vi "TDC_DAQV23_Paralled_muon.vi"(8 "error in (no error)":errorcluster, 9 "stop":bool, 10 "save data":bool=TRUE, 11 "SMA mode":bool) -> (3 "rate":dbl=15.40764551745953)   [LabVIEW 2017]
uses:
  <vilib>/Utility/file.llb/Write Delimited Spreadsheet (DBL).vi
  <vilib>/Utility/file.llb/Write Delimited Spreadsheet (I64).vi
panel:
  out "name (unnamed)":string
  out "x+y":u64
  out "ip":string[](array[string])
  out "error out 4":errorcluster
  in  "timeout (ms) 2":i32=10000
  in  "address":string[](array[string])=["192.168.10.23", "192.168.10.21"]
  out "substring 4":string
  out "substring 3":string
  out "hex integer string":string="07E8"
  out "Year":string="2024"
  out "substring 2":string
  out "substring":string
  in  "factor":i32=128
  in  "displayCR":bool=TRUE
  in  "Counter Setting":dbl=100000.0 format="%#_13g"
  in  "replace dat":bool
  in  "append csv":bool=TRUE
  out "number":u32=23
  out "element":string
  out "fine":u64=375 format="%x"
  in  "UDP Config":bool=TRUE
  in  "data  path":path=path "G:/tdc/2017"
  out "cal 2":u64[](graph)
  in  "Thresholds (mV)":u16[](array[numeric])=[580, 580, 580, 580, 600, 600, 600, 600, 580, 580, 600, 600, 600, 600, 600, 600, 580, 580, 600, 600, 600, 600, 600, 600, 580, 580, 600, 600, 600, 600, 600, 600]
  out "error out 2":errorcluster={"status"=TRUE, "code"=1, "source"="Dequeue Element in TDC_DAQV18_NewStructure.vi"}
  in  "display":bool=TRUE
  in  "Thresholds":u16=580
  in  "one key for threshold":bool=TRUE
  in  "RST":bool
  in  "通道数量":i32=64
  out "Cal Table":u32[](array[numeric])=[33400, 33400, 0, 0, 0, 0, 0, 0, 0, 0, 0, 0, 0, 0, 0, 0, 0, 0, 0, 0, 0, 0, 0, 0, 0, 0, 0, 0, 0, 0, 0, 0, 0, 0, 0, 0, 0, 0, 0, 0, 0, 0, 0, 0, 0, 0, 0, 0, 0, 0, 0, 0, 0, 0, 0, 0, 0, 0, 0, 0, 0, 0, 0, 0]
  in  "channel for cal":i32
  out "channel number":u64=1
  out "Calibration Counter":i32=33403
  out "cal":u32[](graph)=[0, 0, 0, 0, 0, 0, 0, 0, 0, 0, 0, 0, 0, 0, 0, 0, 0, 0, 0, 0, 0, 0, 0, 0, 0, 0, 0, 0, 0, 0, 0, 0, 0, 0, 0, 0, 0, 0, 0, 0, 0, 0, 0, 0, 0, 0, 0, 0, 0, 0, 0, 0, 0, 0, 0, 0, 0, 0, 0, 0, 0, 0, 0, 0, 0, 0, 0, 0, 0, 0, 0, 0, 0, 0, 0, 0, 0, 0, 0, 0, 0, 0, 0, 0, 0, 0, 0, 0, 0, 0, 0, 0, 0, 0, 0, 0, 0, 0, 0, 0, 0, 0, 0, 0, 0, 0, 0, 0, 0, 0, 0, 0, 0, 0, 0, 0, 0, 0, 0, 0, 0, 0, 0, 0, 0, 0, 0, 0, 0, 0, 0, 0, 0, 0, 0, 0, 0, 0, 0, 0, 0, 0, 0, 0, 0, 0, 0, 0, 0, 0, 0, 0, 0, 0, 0, 0, 0, 0, 0, 0, 0, 0, 0, 0, 0, 0, 0, 0, 0, 0, 0, 0, 0, 0, 0, 0, 0, 0, 0, 0, 0, 0, 0, 0, 0, 0, 0, 0, 0, 0, 0, 0, 0, 0, 0, 0, 0, 0, 0, 0, 0, 0, 0, 0, 0, 0, 0, 0, 0, 0, 0, 0, 0, 0, 0, 0, 0, 0, 0, 0, 0, 0, 0, 0, 0, 0, 0, 0, 0, 0, 0, 0, 0, 0, 0, 0, 0, 0, 0, 0, 0, 6, 23, 55, 10, 109, 60, 9, 21, 55, 21, 185, 19, 80, 25, 73, 17, 22, 36, 28, 37, 99, 26, 26, 64, 113, 69, 7, 14, 18, 136, 20, 15, 79, 14, 27, 31, 33, 186, 15, 16, 24, 85, 10, 20, 164, 11, 7, 26, 8, 56, 214, 23, 59, 6, 25, 14, 93, 49, 18, 107, 57, 21, 11, 76, 16, 93, 28, 118, 65, 51, 32, 70, 13, 49, 31, 28, 95, 11, 61, 50, 18, 12, 25, 16, 21, 25, 65, 81, 19, 18, 21, 52, 13, 66, 54, 29, 13, 105, 14, 26, 25, 16, 98, 16, 6, 117, 40, 58, 73, 32, 16, 42, 15, 24, 43, 27, 78, 34, 19, 9, 22, 13, 13, 78, 25, 34, 17, 35, 62, 14, 60, 11, 26, 6, 12, 18, 8, 36, 37, 14, 15, 77, 16, 72, 14, 8, 24, 30, 36, 38, 215, 11, 17, 25, 7, 37, 58, 189, 49, 13, 12, 8, 5, 88, 13, 20, 23, 139, 18, 18, 30, 10, 17, 25, 26, 77, 71, 13, 18, 10, 62, 11, 17, 32, 14, 33, 69, 23, 23, 23, 147, 25, 21, 19, 88, 29, 15, 28, 12, 4, 12, 127, 66, 25, 73, 13, 11, 6, 16, 69, 32, 14, 27, 34, 118, 16, 11, 8, 12, 35, 58, 21, 15, 45, 150, 15, 54, 14, 20, 7, 16, 55, 24, 45, 93, 87, 11, 17, 9, 113, 11, 15, 104, 62, 38, 84, 27, 8, 8, 62, 95, 42, 49, 45, 111, 29, 50, 80, 19, 26, 15, 37, 142, 29, 80, 36, 14, 12, 114, 28, 15, 13, 70, 57, 13, 7, 47, 46, 92, 84, 75, 19, 165, 62, 8, 25, 63, 59, 65, 23, 97, 20, 11, 86, 12, 36, 24, 96, 19, 7, 20, 29, 66, 43, 31, 80, 23, 20, 52, 15, 79, 19, 13, 30, 18, 14, 11, 17, 119, 19, 97, 11, 14, 31, 15, 87, 17, 127, 47, 23, 15, 64, 11, 19, 14, 24, 46, 60, 62, 65, 13, 37, 16, 17, 23, 55, 41, 48, 15, 30, 69, 30, 130, 58, 13, 27, 22, 25, 86, 13, 107, 31, 29, 12, 25, 31, 32, 16, 31, 20, 42, 30, 2, 57, 37, 34, 16, 28, 40, 42, 14, 90, 51, 22, 91, 31, 22, 103, 20, 9, 19, 127, 40, 39, 10, 22, 13, 11, 60, 52, 17, 44, 70, 25, 58, 12, 40, 43, 30, 29, 39, 120, 23, 12, 15, 40, 5, 44, 16, 29, 21, 79, 15, 28, 83, 67, 17, 19, 109, 14, 21, 7, 23, 19, 48, 17, 24, 62, 95, 15, 28, 43, 190, 39, 94, 24, 18, 19, 78, 117, 18, 22, 28, 92, 13, 17, 71, 20, 43, 15, 99, 10, 14, 15, 67, 65, 17, 20, 90, 42, 16, 25, 79, 7, 12, 14, 41, 15, 30, 24, 183, 25, 20, 14, 19, 80, 10, 18, 135, 40, 100, 17, 25, 134, 82, 7, 103, 25, 59, 27, 107, 32, 48, 68, 13, 13, 33, 67, 60, 38, 74, 29, 14, 16, 10, 51, 19, 47, 39, 134, 33, 47, 25, 56, 34, 12, 116, 51, 11, 10, 36, 18, 29, 13, 14, 84, 13, 54, 43, 13, 43, 39, 51, 32, 46, 8, 15, 16, 66, 40, 10, 30, 151, 15, 7, 117, 23, 17, 49, 12, 28, 42, 76, 45, 15, 25, 72, 8, 8, 13, 18, 59, 52, 13, 13, 19, 64, 10, 27, 51, 8, 19, 13, 40, 128, 32, 129, 26, 177, 23, 10, 20, 27, 71, 70, 17, 19, 23, 30, 48, 33, 38, 51, 88, 20, 38, 27, 36, 8, 9, 14, 4, 70, 27, 110, 31, 25, 33, 66, 49, 34, 41, 108, 42, 15, 95, 32, 72, 31, 23, 51, 124, 31, 28, 20, 129, 11, 14, 52, 152, 13, 124, 108, 52, 43, 20, 78, 18, 82, 20, 74, 19, 46, 13, 30, 73, 47, 71, 18, 32, 54, 17, 11, 13, 28, 47, 130, 21, 25, 26, 40, 34, 28, 31, 12, 51, 21, 161, 11, 5, 6, 25, 16, 19, 23, 44, 98, 35, 54, 11, 21, 67, 42, 69, 5, 5, 19, 14, 14, 132, 14, 42, 81, 23, 21, 83, 13, 8, 81, 29, 108, 20, 16, 33, 130, 18, 50, 22, 15, 12, 51, 125, 13, 15, 34, 24, 19, 65, 21, 18, 68, 39, 19, 22, 59, 18, 12, 24, 55, 20, 39, 73, 14, 12, 58, 89, 37, 106, 64, 14, 17, 11, 69, 29, 122, 28, 13, 11, 53, 23, 12, 85, 24, 19, 95, 3, 20, 12, 41, 18, 21, 34, 57, 48, 26, 36, 64, 45, 42, 78, 3, 26, 31, 19, 110, 36, 37, 23, 52, 30, 24, 24, 61, 22, 19, 36, 23, 60, 12, 17, 50, 33, 37, 68, 25, 23, 14, 14, 26, 23, 26, 0, 4, 5, 6, 0, 0, 0, 0, 0, 0, 0, 0, 0, 0, 0, 0, 0, 0, 0, 0, 0, 0, 0, 0, 0, 0, 0, 0, 0, 0, 0, 0, 0, 0, 0, 0, 0, 0, 0, 0, 0, 0, 0, 0, 0, 0, 0, 0, 0, 0, 0, 0, 0, 0, 0, 0, 0, 0, 0, 0, 0, 0, 0, 0, 0, 0, 0, 0, 0, 0, 0, 0, 0, 0, 0, 0, 0, 0, 0, 0, 0, 0, 0, 0, 0, 0, 0, 0, 0, 0, 0, 0, 0, 0, 0, 0, 0, 0, 0, 0, 0, 0, 0, 0, 0, 0, 0, 0, 0, 0, 0, 0, 0, 0, 0, 0, 0, 0, 0, 0, 0, 0, 0, 0, 0, 0, 0, 0, 0, 0, 0, 0, 0, 0, 0, 0, 0, 0, 0, 0, 0, 0, 0, 0, 0, 0, 0, 0, 0, 0, 0, 0, 0, 0, 0, 0, 0, 0, 0, 0, 0, 0, 0, 0, 0, 0, 0, 0, 0, 0, 0, 0, 0, 0, 0, 0, 0, 0, 0, 0, 0, 0, 0, 0, 0, 0, 0, 0, 0, 0, 0, 0, 0, 0, 0, 0, 0, 0, 0, 0, 0, 0, 0, 0, 0, 0, 0, 0, 0, 0, 0, 0, 0, 0, 0, 0, 0, 0, 0, 0, 0, 0, 0, 0, 0, 0, 0, 0, 0, 0, 0, 0, 0, 0, 0, 0, 0, 0, 0, 0, 0, 0, 0, 0, 0, 0, 0, 0, 0, 0, 0, 0, 0, 0, 0, 0, 0, 0, 0, 0, 0, 0, 0, 0, 0, 0, 0, 0, 0, 0, 0, 0, 0, 0, 0, 0, 0, 0, 0, 0, 0, 0, 0, 0, 0, 0, 0, 0, 0, 0, 0, 0, 0, 0, 0, 0, 0, 0, 0, 0, 0, 0, 0, 0, 0, 0, 0, 0, 0, 0, 0, 0, 0, 0, 0, 0, 0, 0, 0, 0, 0, 0, 0, 0, 0, 0, 0, 0, 0, 0, 0, 0, 0, 0, 0, 0, 0, 0, 0, 0, 0, 0, 0, 0, 0, 0, 0, 0, 0, 0, 0, 0, 0, 0, 0, 0, 0, 0, 0, 0, 0, 0, 0, 0, 0, 0, 0, 0, 0, 0, 0, 0, 0, 0, 0, 0, 0, 0, 0, 0, 0, 0, 0, 0, 0, 0, 0, 0, 0, 0, 0, 0, 0, 0, 0, 0, 0, 0, 0, 0, 0, 0, 0, 0, 0, 0, 0, 0, 0, 0, 0, 0, 0, 0, 0, 0, 0, 0, 0, 0, 0, 0, 0, 0, 0, 0, 0, 0, 0, 0, 0, 0, 0, 0, 0, 0, 0, 0, 0, 0, 0, 0, 0, 0, 0, 0, 0, 0, 0, 0, 0, 0, 0, 0, 0, 0, 0, 0, 0, 0, 0, 0, 0, 0, 0, 0, 0, 0, 0, 0, 0, 0, 0, 0, 0, 0, 0, 0, 0, 0, 0, 0, 0, 0, 0, 0, 0, 0, 0, 0, 0, 0, 0, 0, 0, 0, 0, 0, 0, 0, 0, 0, 0, 0, 0, 0, 0, 0, 0, 0, 0, 0, 0, 0, 0, 0, 0, 0, 0, 0, 0, 0, 0, 0, 0, 0, 0, 0, 0, 0, 0, 0, 0, 0, 0, 0, 0, 0, 0, 0, 0, 0, 0, 0, 0, 0, 0, 0, 0, 0, 0, 0, 0, 0, 0, 0, 0, 0, 0, 0, 0, 0, 0, 0, 0, 0, 0, 0, 0, 0, 0, 0, 0, 0, 0, 0, 0, 0, 0, 0, 0, 0, 0, 0, 0, 0, 0, 0, 0, 0, 0, 0, 0, 0, 0, 0, 0, 0, 0, 0, 0, 0, 0, 0, 0, 0, 0, 0, 0, 0, 0, 0, 0, 0, 0, 0, 0, 0, 0, 0, 0, 0, 0, 0, 0, 0, 0, 0, 0, 0, 0, 0, 0, 0, 0, 0, 0, 0, 0, 0, 0, 0, 0, 0, 0, 0, 0, 0, 0, 0, 0, 0, 0, 0, 0, 0, 0, 0, 0, 0, 0, 0, 0, 0, 0, 0, 0, 0, 0, 0, 0, 0, 0, 0, 0, 0, 0, 0, 0, 0, 0, 0, 0, 0, 0, 0, 0, 0, 0, 0, 0, 0, 0, 0, 0, 0, 0, 0, 0, 0, 0, 0, 0, 0, 0, 0, 0, 0, 0, 0, 0, 0, 0, 0, 0, 0, 0, 0, 0, 0, 0, 0, 0, 0, 0, 0, 0, 0, 0, 0, 0, 0, 0, 0, 0, 0, 0, 0, 0, 0, 0, 0, 0, 0, 0, 0, 0, 0, 0, 0, 0, 0, 0, 0, 0, 0, 0, 0, 0, 0, 0, 0, 0, 0, 0, 0, 0, 0, 0, 0, 0, 0, 0, 0, 0, 0, 0, 0, 0, 0, 0, 0, 0, 0, 0, 0, 0, 0, 0, 0, 0, 0, 0, 0, 0, 0, 0, 0, 0, 0, 0, 0, 0, 0, 0, 0, 0, 0, 0, 0, 0, 0, 0, 0, 0, 0, 0, 0, 0, 0, 0, 0, 0, 0, 0, 0, 0, 0, 0, 0, 0, 0, 0, 0, 0, 0, 0, 0, 0, 0, 0, 0, 0, 0, 0, 0, 0, 0, 0, 0, 0, 0, 0, 0, 0, 0, 0, 0, 0, 0, 0, 0, 0, 0, 0, 0, 0, 0, 0, 0, 0, 0, 0, 0, 0, 0, 0, 0, 0, 0, 0, 0, 0, 0, 0, 0, 0, 0, 0, 0, 0, 0, 0, 0, 0, 0, 0, 0, 0, 0, 0, 0, 0, 0, 0, 0, 0, 0, 0, 0, 0, 0, 0, 0, 0, 0, 0, 0, 0, 0, 0, 0, 0, 0, 0, 0, 0, 0, 0, 0, 0, 0, 0, 0, 0, 0, 0, 0, 0, 0, 0, 0, 0, 0, 0, 0, 0, 0, 0, 0, 0, 0, 0, 0, 0, 0, 0, 0, 0, 0, 0, 0, 0, 0, 0, 0, 0, 0, 0, 0, 0, 0, 0, 0, 0, 0, 0, 0, 0, 0, 0, 0, 0, 0, 0, 0, 0, 0, 0, 0, 0, 0, 0, 0, 0, 0]
  out "error out":errorcluster
  out "appended path":path=path "G:/tdc/2017/test_20240929_011527.dat"
  in  "filename":string="test"
  in  "Events":i32=110000 min=1
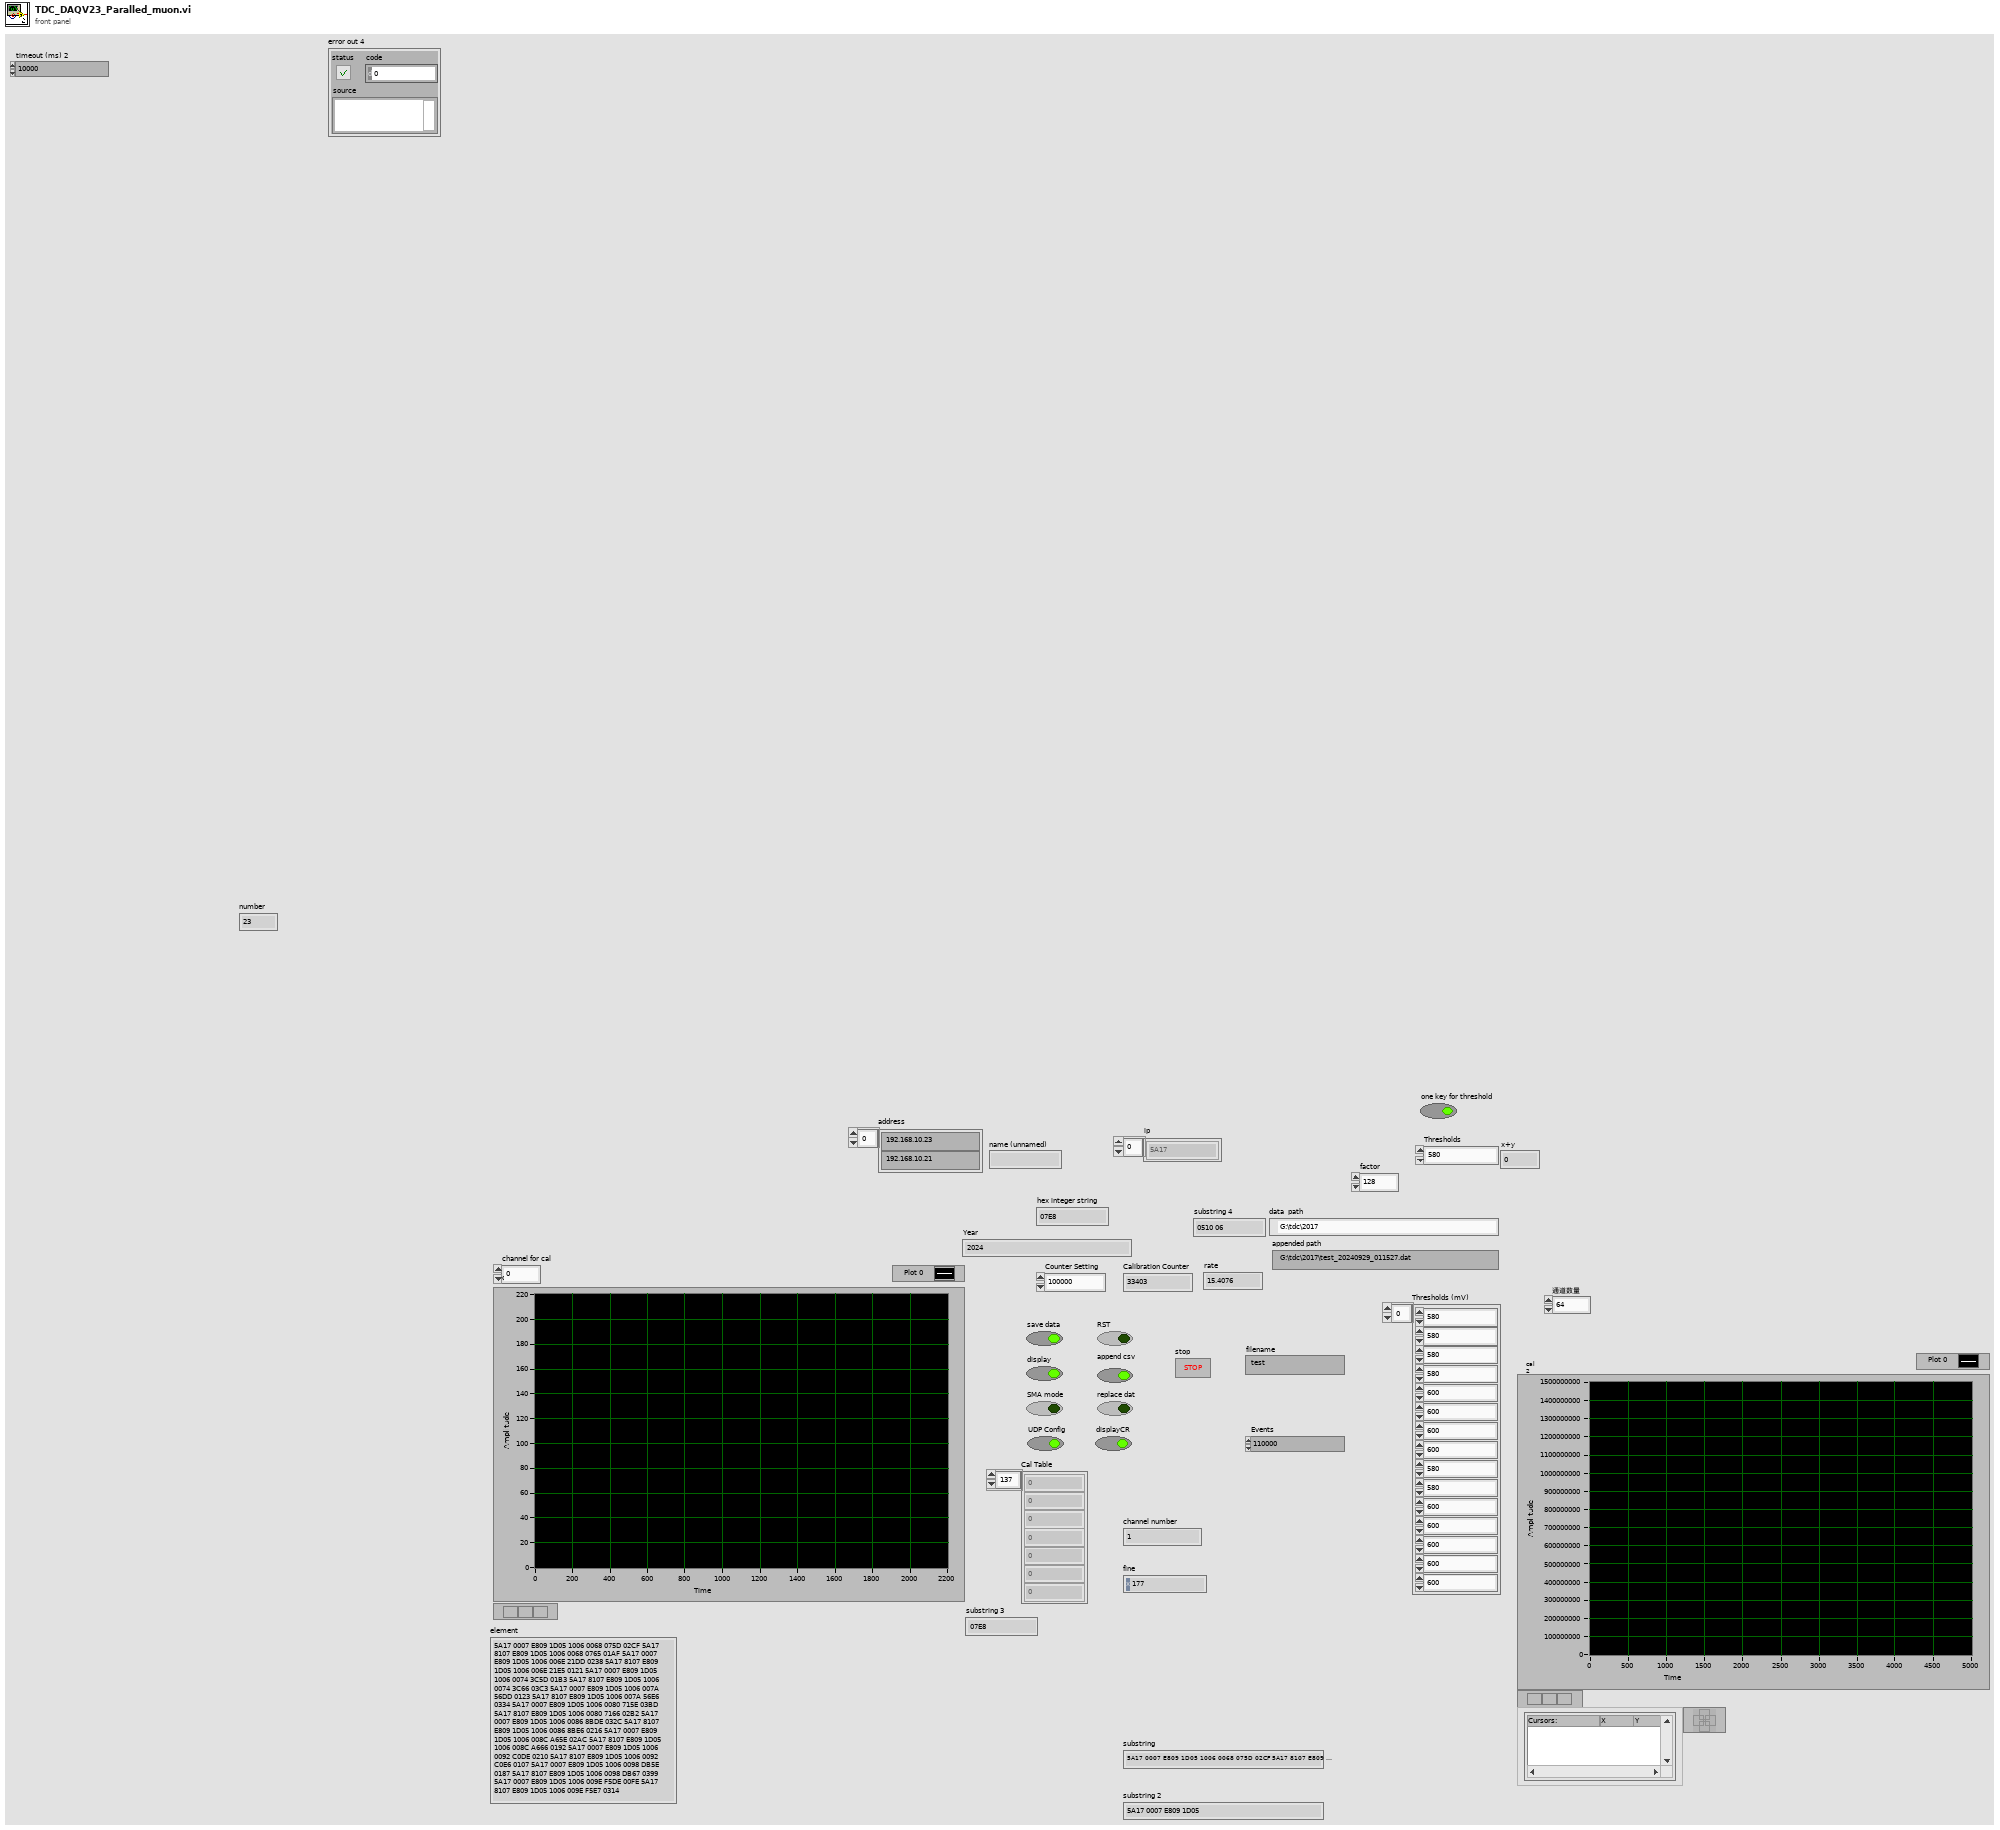
[diagram p1: front panel]
types:
  T1 = enum16{"open", "replace", "create", "open or create", "replace or create", "replace or create with confirmation"}
  T2 = enum16{"big-endian, network order", "native, host order", "little-endian"}
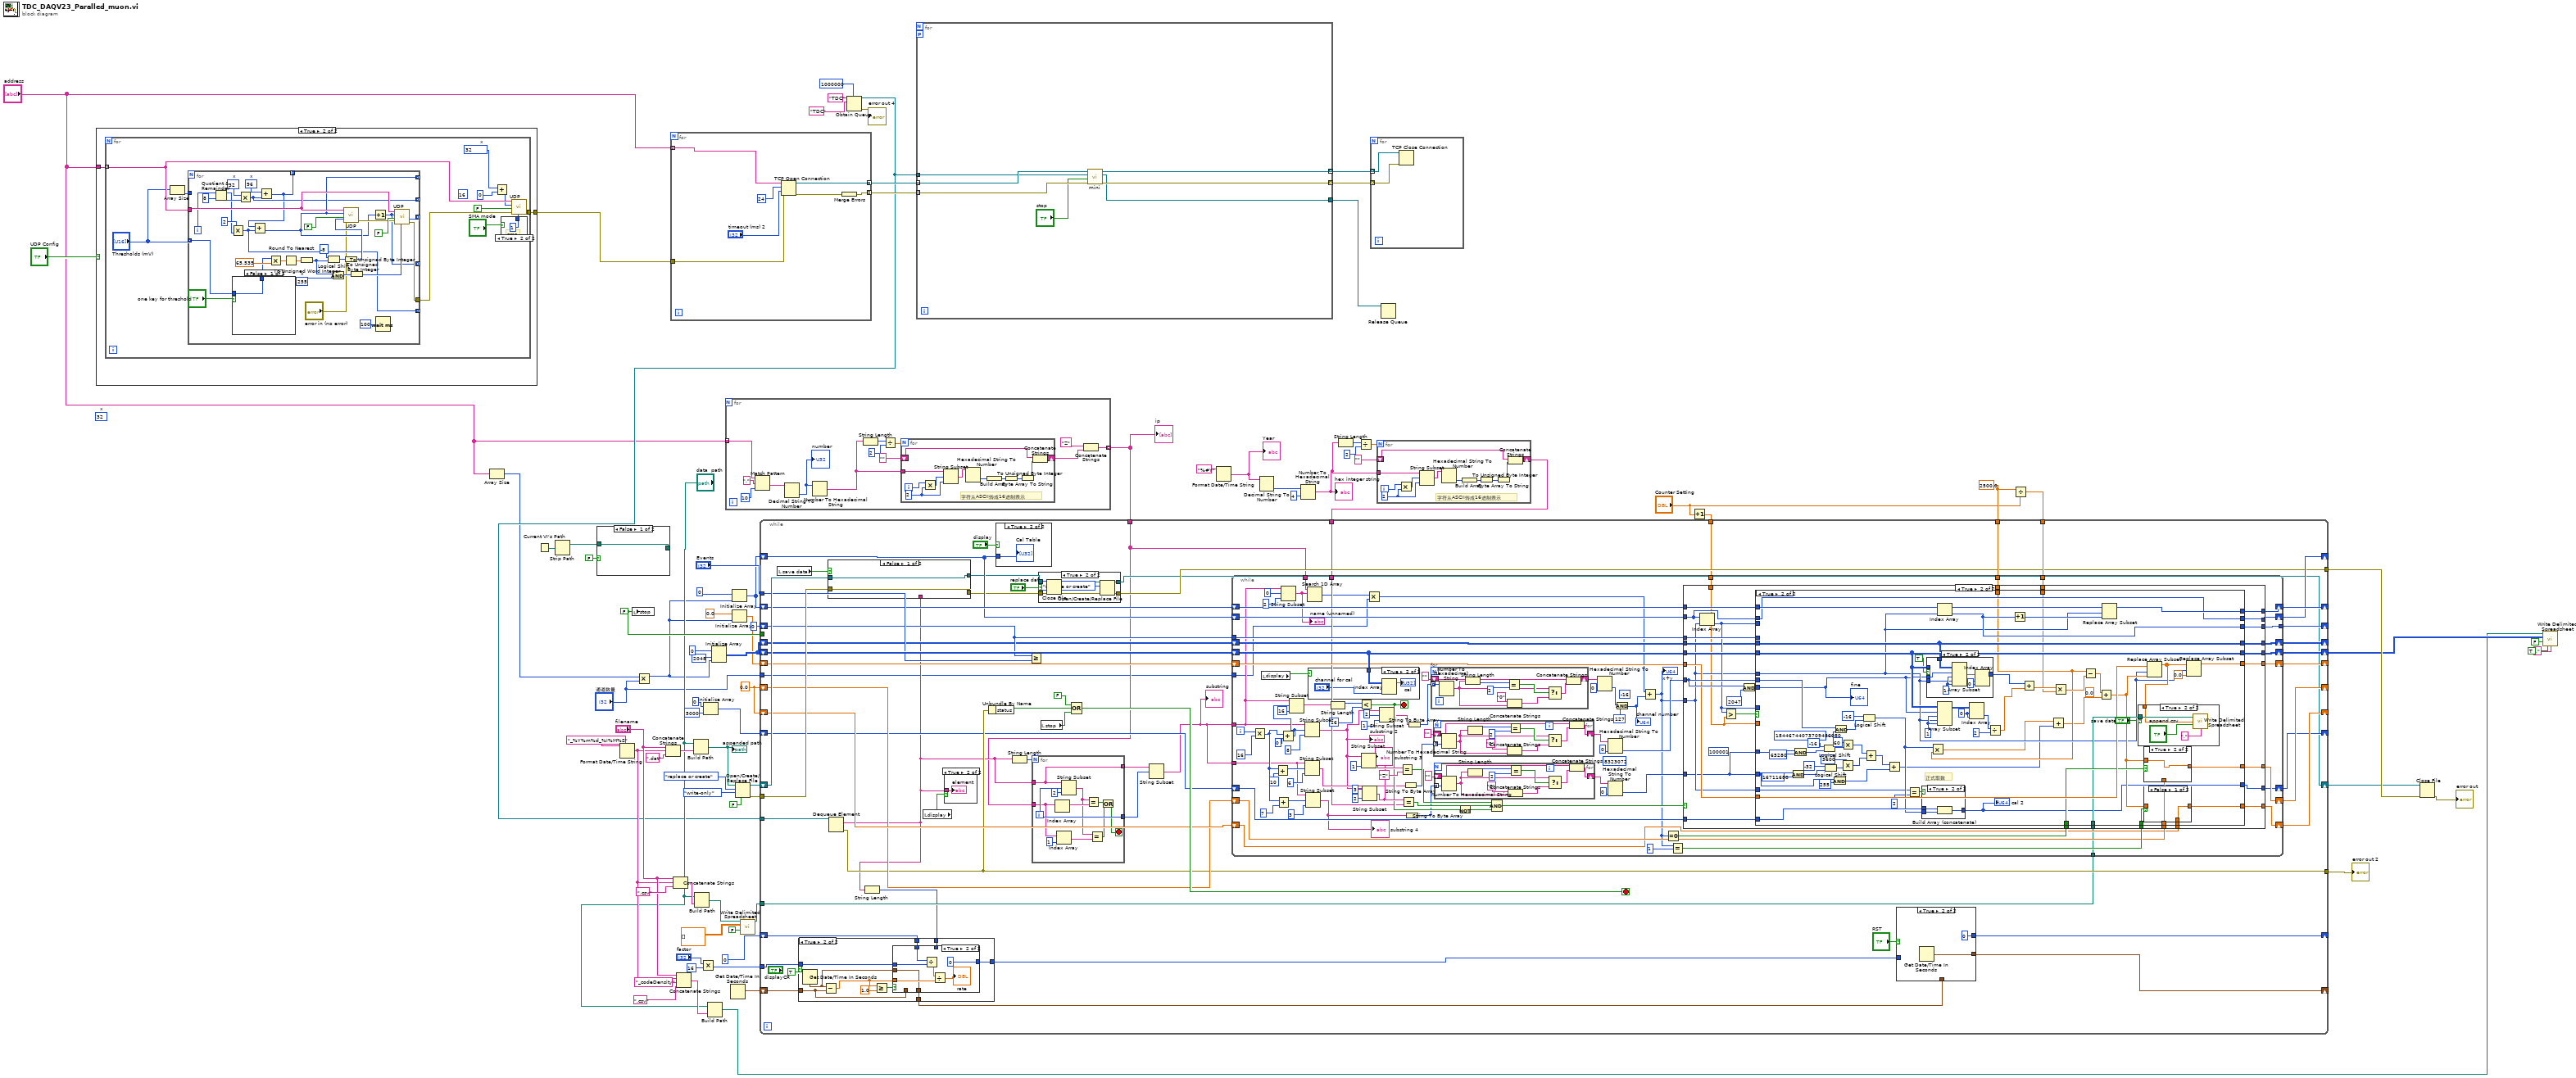
[diagram p0: block diagram]
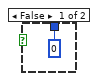
[diagram p3: hidden frame]
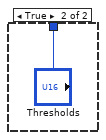
[diagram p4: hidden frame]
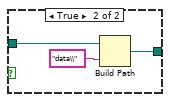
[diagram p5: hidden frame]
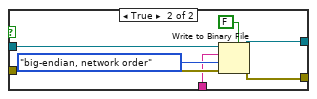
[diagram p7: hidden frame]
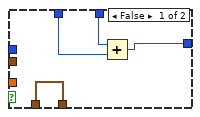
[diagram p10: hidden frame]
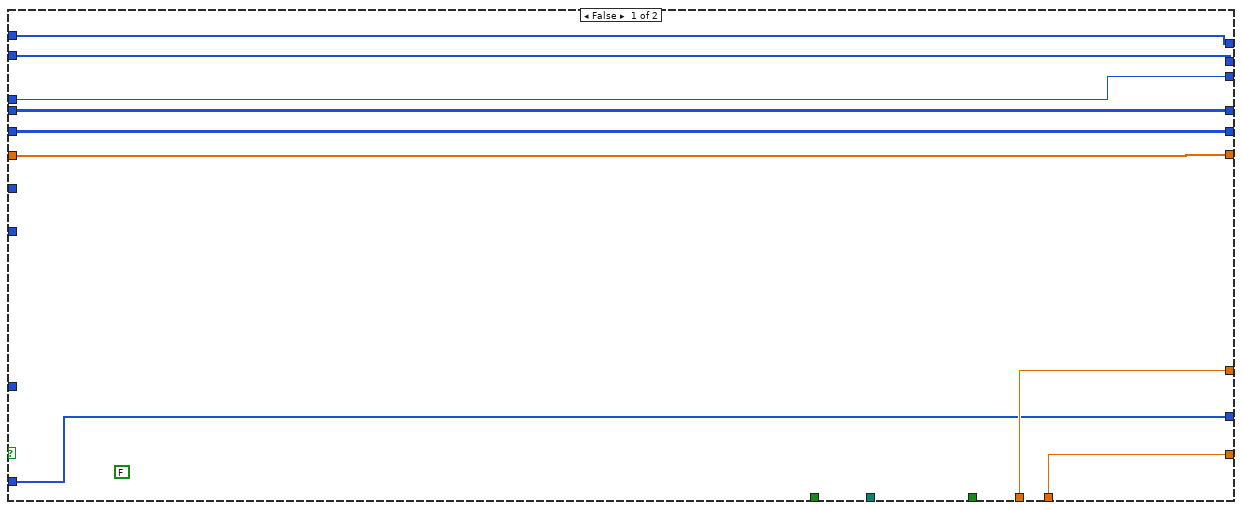
[diagram p14: hidden frame]
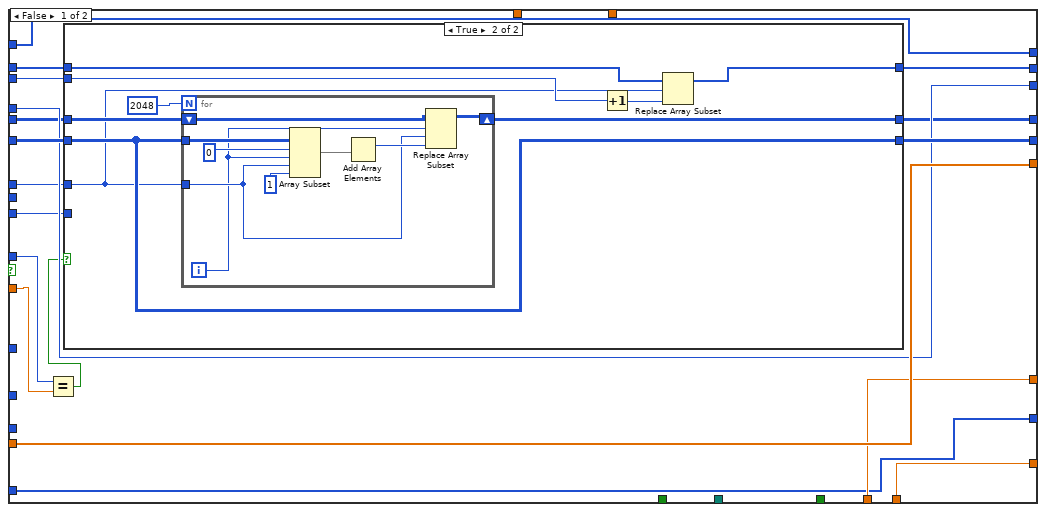
[diagram p15: hidden frame]
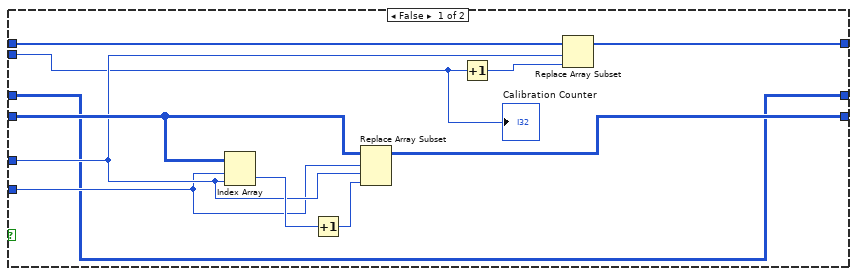
[diagram p16: hidden frame]
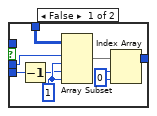
[diagram p19: hidden frame]
diagram:
  w35 = 2500.0 ("x")
  (unwired) u16 32  # x
  w54 = FALSE ("stop")
  w62 = 0.0
  n1 = case shown="True" "UDP Config" {
    tunnel: "address" -> [_ w85]
    tunnel: [_ w84] -> w7
    frame False {
    }
    frame True {
      n2 = for {
        tunnel: w85 -> [w96] mode=indexing
        tunnel: [w93] -> w84
        (unwired) u32 16 ("Address")
        w87 = u16 32  # x
        n3 = Array Size(array="Thresholds (mV)") -> (size(s)=w90:i32)
        n4 = for {
          tunnel: w96 -> [w126]
          tunnel: "Thresholds (mV)" -> [w112] mode=indexing
          tunnel: [w120] -> _ mode=indexing
          tunnel: [w115] -> w94
          tunnel: w90 -> [_]
          tunnel: [w106] -> _ mode=indexing
          tunnel: [w105] -> _ mode=indexing
          tunnel: [w104] -> _ mode=indexing
          tunnel: [w103] -> _ mode=indexing
          tunnel: [w102] -> _ mode=indexing
          i -> [w107]
          w108 = u16 96  # x
          w109 = u16 32  # x
          w122 = u16 255  # x
          n5 = Quotient & Remainder(x=w107, y=8) -> (x-y*floor(x/y)=w101:i32, floor(x/y)=w110:i32)
          n6 = Multiply(x=2, y=w101) -> (x*y=w102:i32)
          n7 = case shown="False" "one key for threshold" {
            tunnel: [w132 "Thresholds"] -> w113
            tunnel: w112 -> [w132 _]
            frame False {
            }
            frame True {
            }
          }
          n8 = Multiply(x=w109, y=w110) -> (x*y=w104:i32)
          n9 = Add(x=w108, y=w104) -> (x+y=w103:i32)
          n10 = Add(x=w103, y=w102) -> (x+y=w106:i32)
          n11 = Multiply(x=w113, y=65.535) -> (x*y=w129:dbl)
          n12 = Round To Nearest(number=w129) -> (nearest integer value=w127:dbl)
          n13 = To Unsigned Word Integer(number=w127) -> (unsigned 16bit integer=w117:u16)
          n14 = Logical Shift(y=i16 -8, x=w117) -> (x << y=w124:u16)
          n15 = And(x=w117, y=w122) -> (x .and. y?=w121:u16)
          n16 = To Unsigned Byte Integer(number=w124) -> (unsigned 8bit integer=w123:u8)
          n17 = call "UDP.vi"("In"=w123, "error in (no error)"="error in (no error)", "Read (TRUE)"=FALSE, "Address"=w106, "IP address"=w126) -> ("error out"=w116:errorcluster)  [unwired: 4 in, 1 out]
          n18 = To Unsigned Byte Integer(number=w121) -> (unsigned 8bit integer=w119:u8)
          n19 = Increment(x=w106) -> (x+1=w105:i32)
          n20 = Wait (ms)(milliseconds to wait=u32 100) -> ()  [unwired: 1 out]
          n21 = call "UDP.vi"("In"=w119, "error in (no error)"=w116, "Read (TRUE)"=FALSE, "Address"=w105, "IP address"=w126) -> ("error out"=w115:errorcluster, "Out"=w120:u8)  [unwired: 4 in]
        }
        n22 = Add(x=w87, y=u32 0 ("Address")) -> (x+y=w86:u32)
        n23 = case shown="True" "SMA mode" {
          tunnel: [u8 0 ("In") u8 1 ("In")] -> w92
          frame False {
          }
          frame True {
            # "sma"
          }
        }
        n24 = call "UDP.vi"("In"=w92, "error in (no error)"=w94, "Read (TRUE)"=FALSE, "Address"=w86, "IP address"=w96) -> ("error out"=w93:errorcluster)  [unwired: 4 in, 1 out]
      }
    }
  }
  n25 = Array Size(array="address") -> (size(s)=w2:i32)
  n26 = Current VI's Path() -> (path=w78:path)
  n27 = Strip Path(path=w78) -> (stripped path=w77:path)  [unwired: 1 out]
  n28 = case shown="False" FALSE {
    tunnel: w77 -> [w134 w136]
    tunnel: [w134 w135] -> _
    frame False {
    }
    frame True {
      n29 = Build Path(base path=w136, name or relative path="data\\") -> (appended path=w135:path)
    }
  }
  n30 = Format Date/Time String(time format string (%c)="_%Y%m%d_%I%M%S") -> (date/time string=w52:string)  [unwired: 2 in]
  n31 = local write "stop"(w54) -> ()
  n32 = Multiply(x=w2, y="通道数量") -> (x*y=w4:i32)
  n33 = Concatenate Strings("filename", w52, ".dat") -> (w76:string)
  n34 = for {
    tunnel: "address" -> [w142] mode=indexing
    tunnel: [w141] -> w16 mode=indexing
    tunnel: [w139] -> w15 mode=indexing
    tunnel: w7 -> [w138]
    n35 = TCP Open Connection(address=w142, remote port or service name=u16 24 ("port"), timeout ms (60000)="timeout (ms) 2", error in (no error)=w138) -> (connection ID=w141:refnum<k5>, error out=w140:errorcluster)  [unwired: 1 in]
    n36 = Merge Errors(w140) -> (w139:errorcluster)
  }
  n37 = Concatenate Strings("filename", w52, ".csv") -> (w64:string)
  n38 = Concatenate Strings("filename", w52, "_codeDensity" ("string"), ".csv") -> (w49:string)
  n39 = Build Path(base path="data  path", name or relative path=w76) -> (appended path=w75:path)
  "appended path" <- w75
  n40 = Build Path(base path="data  path", name or relative path=w64) -> (appended path=w59:path)
  n41 = Multiply(x="factor", y=16) -> (x*y=w28:i32)
  n42 = Initialize Array(u32 0 ("element"), 5000 ("dimension size")) -> (w40:u32[])
  n43 = Build Path(base path="data  path", name or relative path=w49) -> (appended path=w46:path)
  n44 = Initialize Array(u32 0 ("element"), 2048 ("dimension size"), w4) -> (w61:u32[][])
  n45 = for {
    tunnel: [w146] -> w3 mode=indexing
    tunnel: "address" -> [w145] mode=indexing
    n46 = Match Pattern(string=w145, regular expression="." ("search string"), offset (0)=10) -> (after substring=w150:string)  [unwired: 3 out]
    n47 = Decimal String To Number(string=w150) -> (number=w149:i32)  [unwired: 2 in, 1 out]
    "number" <- w149
    n48 = Number To Hexadecimal String(2:w149) -> (0:w148:string)  [unwired: 1 in]
    n49 = String Length(string=w148) -> (length=w155:i32)
    n50 = Divide(x=w155, y=2) -> (x/y=w156:dbl)
    n51 = for {
      N: w156 -> [_]
      shift-right: [w168] -> w147
      shift-left: "" ("format string") -> [w167]
      tunnel: w148 -> [w158]
      i -> [w166]
      w160 = 2 ("y")
      # "字符从ASCII转成16进制表示"
      n52 = Multiply(x=w166, y=w160) -> (x*y=w159:i32)
      n53 = String Subset(string=w158, offset (0)=w159, length (rest)=w160) -> (substring=w161:string)
      n54 = Hexadecimal String To Number(string=w161) -> (number=w165:u32)  [unwired: 2 in, 1 out]
      n55 = Build Array(w165) -> (w164:u32[])
      n56 = To Unsigned Byte Integer(number=w164) -> (unsigned 8bit integer=w163:u8[])
      n57 = Byte Array To String(unsigned byte array=w163) -> (string=w162:string)
      n58 = Concatenate Strings(w167, w162) -> (w168:string)
    }
    n59 = Concatenate Strings("Z", w147) -> (w146:string)
  }
  "ip" <- w3
  n60 = Get Date/Time In Seconds() -> (seconds since 1Jan1904=w55:timestamp)
  n61 = Initialize Array(u32 0 ("element"), w4) -> (w63:u32[])
  n62 = Initialize Array(0.0, w4) -> (w42:dbl[])
  n63 = Open/Create/Replace File(file path (use dialog)=w75, operation (0:open)=T1."replace or create", access (0:read/write)=enum16{"read/write", "read-only", "write-only"}."write-only", disable buffering (F)=FALSE) -> (refnum out=w80:refnum<file>, error out=w79:errorcluster)  [unwired: 2 in, 1 out]
  n64 = call-poly <vilib>:"Write Delimited Spreadsheet.vi"("file path (dialog if empty)"=w59, "2D data"=dbl[][] [], "append to file? (new file:F)"=FALSE) -> ("new file path (Not A Path if cancelled)"=w58:path)  [unwired: 11 in, 1 out]
  n65 = Obtain Queue(max queue size (-1, unlimited)=1000000, name (unnamed)="TDC", element data type="TDC" ("name (unnamed)")) -> (queue out=w6:refnum<queue>, error out=→"error out 4":errorcluster)  [unwired: 2 in, 1 out]
  n66 = for {
    tunnel: w16 -> [w175] mode=indexing
    tunnel: w15 -> [w174] mode=indexing
    tunnel: [w173] -> w14 mode=indexing
    tunnel: [w172] -> w13 mode=indexing
    workers-P: _ -> [_]
    tunnel: w6 -> [w171]
    tunnel: [w170] -> w8
    n67 = call "mini.vi"("error in (no error)"=w174, "stop"="stop", "queue out 2"=w171, "connection ID 2"=w175) -> ("error out 3"=w172:errorcluster, "queue out"=w170:refnum<queue>, "connection ID"=w173:refnum<k5>)  [unwired: 5 in]
  }
  n68 = Format Date/Time String(time format string (%c)="%#Y") -> (date/time string=w25:string)  [unwired: 2 in]
  "Year" <- w25
  n69 = Decimal String To Number(string=w25) -> (number=w24:i32)  [unwired: 2 in, 1 out]
  n70 = Number To Hexadecimal String(1:i16 4 ("width (-)"), 2:w24) -> (0:w18:string)
  "hex integer string" <- w18
  n71 = String Length(string=w18) -> (length=w20:i32)
  n72 = Divide(x=w20, y=2) -> (x/y=w21:dbl)
  n73 = for {
    tunnel: w14 -> [w177] mode=indexing
    tunnel: w13 -> [w176] mode=indexing
    n74 = TCP Close Connection(connection ID=w177, error in (no error)=w176) -> ()  [unwired: 1 in, 2 out]
  }
  n75 = for {
    N: w21 -> [_]
    shift-right: [w188] -> w17
    shift-left: "" ("format string") -> [w187]
    tunnel: w18 -> [w178]
    i -> [w186]
    w180 = 2 ("y")
    # "字符从ASCII转成16进制表示"
    n76 = Multiply(x=w186, y=w180) -> (x*y=w179:i32)
    n77 = String Subset(string=w178, offset (0)=w179, length (rest)=w180) -> (substring=w181:string)
    n78 = Hexadecimal String To Number(string=w181) -> (number=w185:u32)  [unwired: 2 in, 1 out]
    n79 = Build Array(w185) -> (w184:u32[])
    n80 = To Unsigned Byte Integer(number=w184) -> (unsigned 8bit integer=w183:u8[])
    n81 = Byte Array To String(unsigned byte array=w183) -> (string=w182:string)
    n82 = Concatenate Strings(w187, w182) -> (w188:string)
  }
  n83 = Release Queue(queue=w8) -> ()  [unwired: 2 in, 3 out]
  n84 = Increment(x="Counter Setting") -> (x+1=w31:dbl)
  n85 = Divide(x=w35, y="Counter Setting") -> (x/y=w34:dbl)
  n86 = while {
    tunnel: w79 -> [w245]
    tunnel: [w219] -> w43
    tunnel: [w204] -> w72
    shift-right: [w242] -> w47
    shift-left: w61 -> [w243]
    shift-right: [w228] -> _
    shift-left: w42 -> [w241]
    tunnel: "Events" -> [w239]
    shift-right: [w238] -> _
    shift-left: w63 -> [w237]
    shift-right: [w236] -> _
    shift-left: u32 0 ("element") -> [w235]
    shift-right: [w234] -> _
    shift-left: w63 -> [w221]
    shift-right: [w233] -> _
    shift-left: w62 -> [w230]
    shift-right: [w232] -> _
    shift-left: w62 -> [w231]
    shift-right: [w223] -> _
    shift-left: w61 -> [w229]
    tunnel: w58 -> [w215]
    shift-right: [w227] -> _
    shift-left: 0 -> [w198]
    shift-right: [w225] -> _
    shift-left: w55 -> [w224]
    tunnel: w54 -> [_]
    tunnel: w6 -> [w220]
    shift-right: [w216] -> _
    shift-left: w40 -> [w217]
    tunnel: w3 -> [w191]
    tunnel: w35 -> [w210]
    tunnel: w34 -> [w209]
    shift-right: [w203] -> w33
    shift-left: w80 -> [w244]
    tunnel: w31 -> [w202]
    tunnel: w28 -> [w195]
    tunnel: w17 -> [w192]
    tunnel: "通道数量" -> [w190]
    stop <- w240 stop-if-true
    n87 = local read "save data"() -> (w197:bool)
    n88 = Dequeue Element(queue=w220) -> (element=w208:string, error out=w219:errorcluster)  [unwired: 2 in, 2 out]
    n89 = case shown="False" w197 {
      tunnel: w245 -> [w247 w255]
      tunnel: w244 -> [w248 w254]
      tunnel: w208 -> [_ w251]
      tunnel: [w248 w250] -> w207
      tunnel: [w247 w249] -> w205
      frame False {
      }
      frame True {
        n90 = Write to Binary File(file (use dialog)=w254, data=w251, error in=w255, 5:FALSE ("prepend array or string size? (T)"), 9:T2."big-endian, network order" ("byte order (0:big-endian, network order)")) -> (refnum out=w250:refnum<file>, error out=w249:errorcluster)  [unwired: 1 in, 1 out]
      }
    }
    n91 = String Length(string=w208) -> (length=w199:i32)
    n92 = case shown="True" TRUE {
      tunnel: w224 -> [w277 w282]
      tunnel: [w277 w283] -> w201
      tunnel: w198 -> [w276 w281]
      tunnel: w199 -> [_ w280]
      tunnel: [w276 w279] -> w200
      tunnel: w195 -> [_ w278]
      frame False {
      }
      frame True {
        n93 = Get Date/Time In Seconds() -> (seconds since 1Jan1904=w284:timestamp)
        n94 = Subtract(x=w284, y=w282) -> (x-y=w286:dbl)
        n95 = Greater Or Equal?(x=w286, y=1.0) -> (x >= y?=w287:bool)
        n96 = case shown="True" w287 {
          tunnel: w286 -> [_ w298]
          tunnel: w284 -> [_ w296]
          tunnel: [w291 w296] -> w283
          tunnel: w282 -> [w291 _]
          tunnel: w281 -> [w290 w293]
          tunnel: w280 -> [w289 _]
          tunnel: [w288 0] -> w279
          tunnel: w278 -> [_ w292]
          frame False {
            n97 = Add(x=w289, y=w290) -> (x+y=w288:i32)
          }
          frame True {
            n98 = Divide(x=w293, y=w292) -> (x/y=w295:dbl)
            n99 = Divide(x=w295, y=w298) -> (x/y=→"rate":dbl)
          }
        }
      }
    }
    n100 = local read "display"() -> (w196:bool)
    n101 = case shown="True" w196 {
      tunnel: w208 -> [_ w246]
      frame False {
      }
      frame True {
        "element" <- w246
      }
    }
    n102 = Unbundle By Name(w219) -> ("status"=w218:bool)
    n103 = case shown="True" "display" {
      tunnel: w221 -> [_ w299]
      frame False {
      }
      frame True {
        "Cal Table" <- w299
      }
    }
    n104 = String Length(string=w208) -> (length=w214:i32)
    n105 = Greater Or Equal?(x=w235, y=w239) -> ()  [unwired: 1 out]
    n106 = for {
      N: w214 -> [_]
      tunnel: w208 -> [w273]
      tunnel: [w273] -> w213
      tunnel: [w272] -> w212
      tunnel: w191 -> [w270]
      i -> [w272]
      stop <- w266 stop-if-true
      n107 = Index Array(array=w270) -> (element=w271:string)  [unwired: 1 in]
      n108 = Index Array(array=w270, index=1) -> (element=w268:string)
      n109 = String Subset(string=w273, offset (0)=w272, length (rest)=2 ("length (rest)")) -> (substring=w267:string)
      n110 = Equal?(x=w267, y=w271) -> (x = y?=w274:bool)
      n111 = Equal?(x=w267, y=w268) -> (x = y?=w265:bool)
      n112 = Or(x=w274, y=w265) -> (x .or. y?=w266:bool)
    }
    n113 = case shown="True" "replace dat" {
      tunnel: w207 -> [w257 w263]
      tunnel: [w257 w262] -> w203
      tunnel: w205 -> [w256 w259]
      tunnel: [w256 w258] -> w204
      frame False {
      }
      frame True {
        n114 = Close File(refnum=w263, error in=w259) -> (path=w264:path, error out=w260:errorcluster)
        n115 = Open/Create/Replace File(file path (use dialog)=w264, error in=w260, operation (0:open)=T1."replace or create") -> (refnum out=w262:refnum<file>, error out=w258:errorcluster)  [unwired: 3 in, 1 out]
      }
    }
    n116 = local read "stop"() -> (w189:bool)
    n117 = Compound Arithmetic op=OR(FALSE ("x"), w218, w189) -> (w240:bool)
    n118 = String Subset(string=w213, offset (0)=w212) -> (substring=w193:string)  [unwired: 1 in]
    "substring" <- w193
    n119 = while {
      tunnel: w193 -> [w311]
      shift-right: [w386] -> w242
      shift-left: w243 -> [w384]
      shift-right: [w382] -> w228
      shift-left: w241 -> [w383]
      shift-right: [w379] -> w238
      shift-left: w237 -> [w378]
      tunnel: [w377] -> w236
      tunnel: w235 -> [w376]
      shift-right: [w374] -> w234
      shift-left: w221 -> [w375]
      shift-right: [w370] -> w233
      shift-left: w230 -> [w368]
      shift-right: [w366] -> w232
      shift-left: w231 -> [w367]
      tunnel: w215 -> [w365]
      shift-right: [w364] -> w223
      shift-left: w229 -> [w333]
      shift-right: [w361] -> w216
      shift-left: w217 -> [w362]
      tunnel: w193 -> [w325]
      tunnel: w210 -> [w340]
      tunnel: w209 -> [w339]
      tunnel: w202 -> [w332]
      tunnel: w192 -> [w319]
      tunnel: w191 -> [w310]
      tunnel: w190 -> [w307]
      i -> [w387]
      stop <- w335 stop-if-true
      (unwired) u64 8323072 ("port")
      (unwired) i16 -16 ("y")
      n120 = Multiply(x=w387, y=16 ("length (rest)")) -> (x*y=w326:i32)
      n121 = local read "display"() -> (w363:bool)
      n122 = Add(x=w326, y=10 ("length (rest)")) -> (x+y=w353:i32)
      n123 = Add(x=w326, y=7 ("length (rest)")) -> (x+y=w328:i32)
      n124 = String Subset(string=w311, offset (0)=0, length (rest)=2 ("length (rest)")) -> (substring=w304:string)
      "name (unnamed)" <- w304
      n125 = Add(x=w326, y=0 ("length (rest)")) -> (x+y=w338:i32)
      n126 = String Subset(string=w311, offset (0)=w338, length (rest)=16 ("y")) -> (substring=w336:string)
      n127 = String Subset(string=w311, offset (0)=w338, length (rest)=8 ("length (rest)")) -> (substring=w317:string)
      "substring 2" <- w317
      n128 = String Subset(string=w325, offset (0)=w353, length (rest)=6 ("length (rest)")) -> (substring=w331:string)
      n129 = String Subset(string=w325, offset (0)=w328, length (rest)=3 ("length (rest)")) -> (substring=w314:string)
      "substring 4" <- w314
      n130 = Search 1D Array(1D array=w310, element=w304) -> (index of element=w308:i32)  [unwired: 1 in]
      n131 = case shown="True" w363 {
        tunnel: w384 -> [_ w413]
        frame False {
        }
        frame True {
          n132 = Index Array(array=w413, index (col)="channel for cal") -> (element=→"cal":u32[])  [unwired: 1 in]
        }
      }
      n133 = String Length(string=w336) -> (length=w381:i32)
      n134 = Less?(x=w381, y=16) -> (x < y?=w335:bool)
      n135 = String Subset(string=w317, length (rest)=1 ("length (rest)")) -> (substring=w358:string)  [unwired: 1 in]
      n136 = String Subset(string=w317, offset (0)=3, length (rest)=2 ("length (rest)")) -> (substring=w341:string)
      "substring 3" <- w341
      n137 = Multiply(x=w308, y=w307) -> (x*y=w306:i32)
      n138 = String Subset(string=w317, offset (0)=2, length (rest)=1 ("length (rest)")) -> (substring=w315:string)
      n139 = Equal?(x=w358, y="Z" ("format string")) -> (x = y?=w343:bool)
      n140 = Equal?(x=w341, y=w319) -> (x = y?=w342:bool)
      n141 = String To Byte Array(string=w331) -> (unsigned byte array=w350:u8[])
      n142 = String To Byte Array(string=w314) -> (unsigned byte array=w321:u8[])
      n143 = String To Byte Array(string=w315) -> (unsigned byte array=w389:u8[])
      n144 = for {
        shift-right: [w601] -> w347
        shift-left: "" ("format string") -> [w598]
        tunnel: w389 -> [w602] mode=indexing
        n145 = Number To Hexadecimal String(2:w602) -> (0:w594:string)  [unwired: 1 in]
        n146 = String Length(string=w594) -> (length=w600:i32)
        n147 = Equal?(x=w600, y=2) -> (x = y?=w597:bool)
        n148 = Concatenate Strings("0" ("format string"), w594) -> (w596:string)
        n149 = Select(t=w594, s=w597, f=w596) -> (s? t:f=w593:string)
        n150 = Concatenate Strings(w598, w593) -> (w601:string)
      }
      n151 = for {
        shift-right: [w409] -> w348
        shift-left: "" ("format string") -> [w401]
        tunnel: w350 -> [w410] mode=indexing
        n152 = Number To Hexadecimal String(2:w410) -> (0:w403:string)  [unwired: 1 in]
        n153 = String Length(string=w403) -> (length=w408:i32)
        n154 = Concatenate Strings("0" ("format string"), w403) -> (w405:string)
        n155 = Equal?(x=w408, y=2) -> (x = y?=w406:bool)
        n156 = Select(t=w403, s=w406, f=w405) -> (s? t:f=w402:string)
        n157 = Concatenate Strings(w401, w402) -> (w409:string)
      }
      n158 = for {
        shift-right: [w399] -> w324
        shift-left: "" ("format string") -> [w391]
        tunnel: w321 -> [w400] mode=indexing
        n159 = Number To Hexadecimal String(2:w400) -> (0:w393:string)  [unwired: 1 in]
        n160 = String Length(string=w393) -> (length=w398:i32)
        n161 = Concatenate Strings("0" ("format string"), w393) -> (w395:string)
        n162 = Equal?(x=w398, y=2) -> (x = y?=w396:bool)
        n163 = Select(t=w393, s=w396, f=w395) -> (s? t:f=w392:string)
        n164 = Concatenate Strings(w391, w392) -> (w399:string)
      }
      n165 = Not(x=w335) -> (.not. x?=w334:bool)
      n166 = Compound Arithmetic op=AND(w343, w342, w334) -> (w356:bool)
      n167 = Hexadecimal String To Number(string=w347, default (0uL)=u64 0 ("default (0 U32)")) -> (number=w385:u64)  [unwired: 1 in, 1 out]
      n168 = Hexadecimal String To Number(string=w348, default (0uL)=u64 0 ("default (0 U32)")) -> (number=w346:u64)  [unwired: 1 in, 1 out]
      n169 = Hexadecimal String To Number(string=w324, default (0uL)=u64 0 ("default (0 U32)")) -> (number=w320:u64)  [unwired: 1 in, 1 out]
      n170 = And(x=w385, y=u64 127 ("port")) -> (x .and. y?=w309:u64)
      "channel number" <- w309
      n171 = Add(x=w306, y=w309) -> (x+y=w305:u64)
      "x+y" <- w305
      n172 = Equal To 0?(x=w305) -> (x = 0?=w371:bool)
      n173 = Equal?(x=w305, y=u64 1) -> (x = y?=w369:bool)
      n174 = case shown="True" w356 {
        tunnel: w346 -> [_ w453]
        tunnel: w376 -> [w419 w443]
        tunnel: w384 -> [w422 w452]
        tunnel: [w422 w451] -> w386
        tunnel: [w421 w448] -> w382
        tunnel: w383 -> [w421 w447]
        tunnel: w305 -> [_ w427]
        tunnel: w378 -> [w420 w446]
        tunnel: [w420 w445] -> w379
        tunnel: [w419 w444] -> w377
        tunnel: w375 -> [w418 w442]
        tunnel: [w418 w441] -> w374
        tunnel: w371 -> [_ w440]
        tunnel: w368 -> [w417 w439]
        tunnel: [w417 w438] -> w370
        tunnel: w369 -> [_ w437]
        tunnel: w367 -> [w416 w436]
        tunnel: [w416 w435] -> w366
        tunnel: w333 -> [w415 w433]
        tunnel: [w415 w432] -> w364
        tunnel: w365 -> [_ w431]
        tunnel: w362 -> [w414 w429]
        tunnel: [w414 w428] -> w361
        tunnel: w340 -> [_ w426]
        tunnel: w339 -> [_ w425]
        tunnel: w332 -> [_ w424]
        tunnel: w320 -> [_ w423]
        frame False {
          (unwired) FALSE
        }
        frame True {
          (unwired) 100001 ("y")
          n175 = Index Array(array=w442, index=w427) -> (element=w434:u32)
          n176 = Greater?(x=w434, y=w424) -> (0:w430:bool)
          n177 = And(x=w453, y=u64 2047 ("port")) -> (x .and. y?=w449:u64)
          n178 = case shown="True" w430 {
            tunnel: w453 -> [_ w565]
            tunnel: w452 -> [w471 w551]
            tunnel: [w470 w551] -> w451
            tunnel: w449 -> [w462 w524]
            tunnel: [w469 w535] -> w448
            tunnel: w447 -> [w469 w558]
            tunnel: w443 -> [w467 _]
            tunnel: w427 -> [w465 w533]
            tunnel: w446 -> [w468 w557]
            tunnel: [w468 w556] -> w445
            tunnel: [w467 w554] -> w444
            tunnel: w434 -> [w463 _]
            tunnel: w442 -> [w466 w553]
            tunnel: [w464 w553] -> w441
            tunnel: w440 -> [_ w546]
            tunnel: w439 -> [w461 w545]
            tunnel: [w461 w544] -> w438
            tunnel: w437 -> [_ w543]
            tunnel: w436 -> [w460 w542]
            tunnel: [w460 w541] -> w435
            tunnel: w434 -> [w458 _]
            tunnel: w424 -> [w455 _]
            tunnel: w433 -> [w457 w537]
            tunnel: [w456 w537] -> w432
            tunnel: w431 -> [_ w536]
            tunnel: w429 -> [w454 w530]
            tunnel: [w454 w528] -> w428
            tunnel: w427 -> [_ w525]
            tunnel: w426 -> [_ w522]
            tunnel: w425 -> [_ w523]
            tunnel: w423 -> [_ w517]
            tunnel: w423 -> [_ w505]
            frame False {
              n179 = Equal?(x=w458, y=w455) -> (x = y?=w459:bool)
              n180 = case shown="True" w459 {
                tunnel: w471 -> [w482 w488]
                tunnel: [w480 w488] -> w470
                tunnel: w466 -> [w478 w486]
                tunnel: w465 -> [w477 w483]
                tunnel: [w475 w485] -> w464
                tunnel: w463 -> [w474 w484]
                tunnel: w462 -> [w473 _]
                tunnel: w457 -> [w472 w490]
                tunnel: [w472 w489] -> w456
                frame False {
                  n181 = Index Array(array=w482, index (row)=w473, index (col)=w477) -> (element=w481:u32)
                  n182 = Increment(x=w481) -> (x+1=w479:u32)
                  n183 = Replace Array Subset(array=w482, new element=w479, index (row)=w473, index (col)=w477) -> (w480:u32[][])
                  n184 = Increment(x=w474) -> (x+1=w476:u32)
                  n185 = Replace Array Subset(array=w478, new element=w476, index=w477) -> (w475:u32[])
                  "Calibration Counter" <- w474
                }
                frame True {
                  n186 = for {
                    N: 2048 -> [_]
                    tunnel: w488 -> [w500]
                    tunnel: w483 -> [w493]
                    shift-right: [w495] -> w489
                    shift-left: w490 -> [w496]
                    i -> [w492]
                    n187 = Array Subset(array=w500, index (row)=0 ("索引"), length (row)=w492, index (col)=w493, length (col)=1 ("长度")) -> (w497:u32[][])
                    n188 = Add Array Elements(numeric array=w497) -> (sum=w494:u32)
                    n189 = Replace Array Subset(array=w496, new element=w494, index (row)=w492, index (col)=w493) -> (w495:u32[][])
                  }
                  n190 = Increment(x=w484) -> (x+1=w487:u32)
                  n191 = Replace Array Subset(array=w486, new element=w487, index=w483) -> (w485:u32[])
                }
              }
            }
            frame True {
              (unwired) 0.0 ("x")
              w548 = 0 ("索引 (行)")
              w550 = 1 ("长度")
              # "正式取数"
              n192 = And(x=w505, y=u64 16711680 ("port")) -> (x .and. y?=w514:u64)
              n193 = And(x=w517, y=u64 65280 ("port")) -> (x .and. y?=w520:u64)
              n194 = Logical Shift(y=i16 -16, x=w520) -> (x << y=w511:u64)
              n195 = Logical Shift(y=i16 -32, x=w514) -> (x << y=w513:u64)
              n196 = And(x=w505, y=u64 255 ("port")) -> (x .and. y?=w504:u64)
              n197 = And(x=w565, y=u64 18446744073709486080 ("port")) -> (x .and. y?=w562:u64)
              n198 = Multiply(x=u64 3600, y=w513) -> (x*y=w508:u64)
              n199 = Multiply(x=u64 60, y=w511) -> (x*y=w509:u64)
              n200 = Logical Shift(y=i16 -16, x=w562) -> (x << y=w529:u64)
              n201 = Add(x=w509, y=w508) -> (x+y=w507:u64)
              n202 = Add(x=w507, y=w504) -> (x+y=w501:u64)
              n203 = Equal?(x=w525, y=u32 2) -> (x = y?=w527:bool)
              n204 = case shown="True" w527 {
                tunnel: w530 -> [w566 w569]
                tunnel: w529 -> [_ w568]
                tunnel: [w566 w567] -> w528
                frame False {
                }
                frame True {
                  n205 = Build Array (concatenate)(w569, w568) -> (w567:u64[])
                }
              }
              "cal 2" <- w528
              n206 = case shown="True" TRUE {
                tunnel: [w576 w584] -> w560
                tunnel: w551 -> [_ _]
                tunnel: w533 -> [w581 w582]
                tunnel: w524 -> [w579 w587]
                tunnel: w537 -> [w580 w588]
                frame False {
                  w575 = 0 ("index (row)")
                  w578 = 1 ("长度")
                  n207 = Decrement(x=w581) -> (x-1=w574:u64)
                  n208 = Array Subset(array=w580, index (row)=w579, length (row)=w578, index (col)=w574, length (col)=w578) -> (w577:u32[][])
                  n209 = Index Array(array=w577, index (row)=w575, index (col)=w575) -> (element=w576:u32)
                }
                frame True {
                  w583 = 0 ("index (row)")
                  w586 = 1 ("长度")
                  n210 = Array Subset(array=w588, index (row)=w587, length (row)=w586, index (col)=w582, length (col)=w586) -> (w585:u32[][])
                  n211 = Index Array(array=w585, index (row)=w583, index (col)=w583) -> (element=w584:u32)
                }
              }
              n212 = Multiply(x=w529, y=w522) -> (x*y=w503:dbl)
              n213 = Index Array(array=w557, index=w533) -> (element=w554:u32)
              n214 = Array Subset(array=w551, index (row)=w524, length (row)=w550, index (col)=w533, length (col)=w550) -> (w549:u32[][])
              n215 = Index Array(array=w549, index (row)=w548, index (col)=w548) -> (element=w547:u32)
              n216 = Divide(x=w547, y=u32 2) -> (x/y=w552:dbl)
              n217 = Increment(x=w554) -> (x+1=w555:u32)
              n218 = Add(x=w560, y=w552) -> (x+y=w559:dbl)
              n219 = Add(x=w503, y=w501) -> (x+y=w502:dbl)
              n220 = Multiply(x=w559, y=w523) -> (x*y=w539:dbl)
              n221 = Subtract(x=w522, y=w539) -> (x-y=w521:dbl)
              n222 = Add(x=w521, y=w502) -> (x+y=w540:dbl)
              n223 = Replace Array Subset(array=w557, new element=w555, index=w533) -> (w556:u32[])
              n224 = case shown="True" w546 {
                tunnel: w540 -> [_ w592]
                tunnel: [w591 w592] -> w544
                tunnel: w545 -> [w591 _]
                frame False {
                }
                frame True {
                }
              }
              n225 = case shown="False" w543 {
                tunnel: [w589 w590] -> w541
                tunnel: w542 -> [w589 _]
                tunnel: w540 -> [_ w590]
                frame False {
                }
                frame True {
                }
              }
              n226 = Replace Array Subset(array=w558, new element=w540, index=w533) -> (w534:dbl[])
              n227 = case shown="True" "save data" {
                tunnel: w536 -> [_ w573]
                tunnel: w534 -> [_ w571]
                frame False {
                }
                frame True {
                  n228 = call-poly <vilib>:"Write Delimited Spreadsheet.vi"("file path (dialog if empty)"=w573, "1D data"=w571, "append to file? (new file:F)"="append csv", "delimiter (\\t)"="," ("delimiter (\\t)")) -> ()  [unwired: 10 in, 2 out]
                }
              }
              n229 = Replace Array Subset(array=w534, new element=0.0 ("new element/subarray"), index=w533) -> (w535:dbl[])
              "fine" <- w524
            }
          }
        }
      }
    }
    n230 = case shown="True" "RST" {
      tunnel: w200 -> [w301 _]
      tunnel: [w301 0] -> w227
      tunnel: [w300 w302] -> w225
      tunnel: w201 -> [w300 _]
      frame False {
      }
      frame True {
        n231 = Get Date/Time In Seconds() -> (seconds since 1Jan1904=w302:timestamp)
      }
    }
  }
  "error out 2" <- w43
  n232 = Close File(refnum=w33, error in=w72) -> (error out=→"error out":errorcluster)  [unwired: 1 out]
  n233 = call-poly <vilib>:"Write Delimited Spreadsheet.vi"("file path (dialog if empty)"=w46, "2D data"=w47, "append to file? (new file:F)"=FALSE, "transpose? (no:F)"=TRUE, "delimiter (\\t)"="," ("delimiter (\\t)")) -> ()  [unwired: 9 in, 2 out]
